vi "Connect.vi"(6 "Local Data":T1, 8 "error in":errorcluster) -> (0 "error out":errorcluster, 4 "Local Data Out":T1)   [LabVIEW 2025, in "Instrument B.lvlib"]
uses:
  Controls/Local Data_Acquisition.ctl
  Instrument B.lvlib
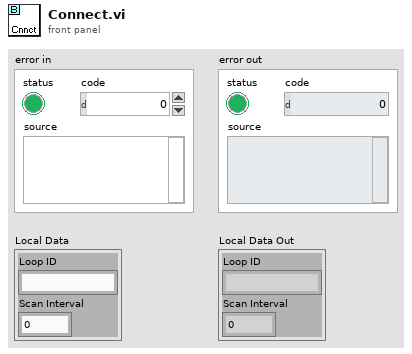
[diagram p1: front panel]
types:
  T1 = typedef "Local Data_Acquisition.ctl" = cluster{"Loop ID":string, "Scan Interval":u32}
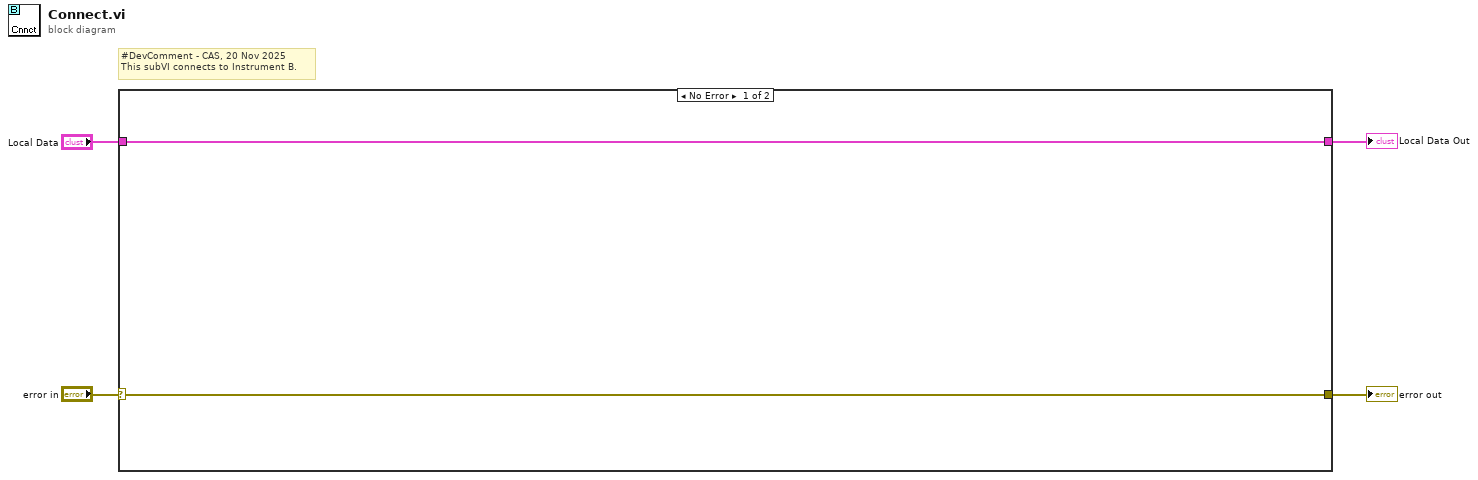
[diagram p0: block diagram]
diagram:
  # "#DevComment - CAS, 20 Nov 2025\nThis subVI connects to Instrument B."
  n1 = case shown="No Error" "error in" {
    selector: "error in" -> [w6 w8]
    tunnel: [w6 w8] -> w3
    tunnel: [w5 w7] -> w2
    tunnel: "Local Data" -> [w5 w7]
    frame No Error {
    }
    frame Error {
    }
  }
  "error out" <- w3
  "Local Data Out" <- w2
